vi "스테이트머신_계측기(간단).vi"() -> ()   [LabVIEW 2020]
panel:
  out "열거형":enum16{"초기", "대기", "계측"}(ring)
  out "진도":dbl(graph)
  in  "계측 시작":bool
  in  "프로그램 정지":bool
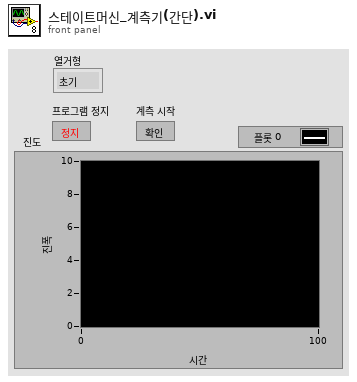
[diagram p1: front panel]
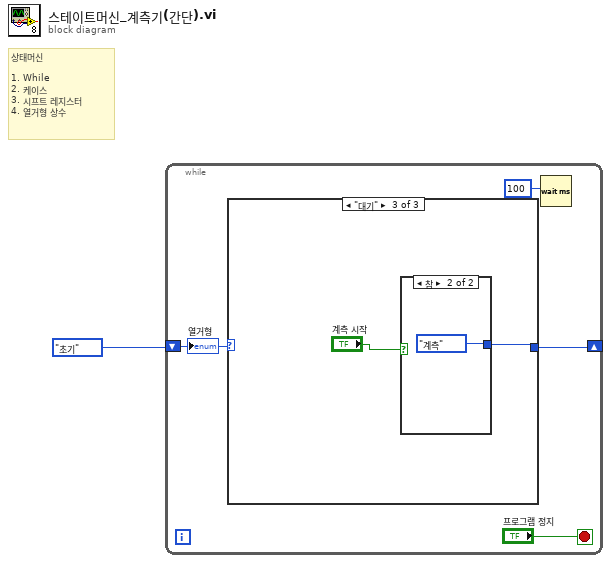
[diagram p0: block diagram]
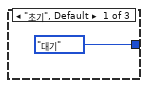
[diagram p2: hidden frame]
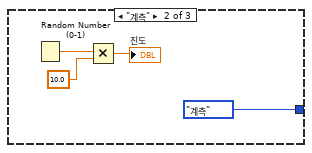
[diagram p3: hidden frame]
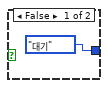
[diagram p4: hidden frame]
diagram:
  # "상태머신\n\n1. While\n2. 케이스 \n3. 시프트 레지스터\n4. 열거형 상수"
  n1 = while {
    shift-right: [w2] -> _
    shift-left: enum16{"초기", "대기", "계측"}."초기" -> [w4]
    stop <- "프로그램 정지" stop-if-true
    n2 = case shown="\"대기\"" w4 {
      tunnel: [enum16{"초기", "대기", "계측"}."대기" enum16{"초기", "대기", "계측"}."계측" w11] -> w2
      frame "초기", Default {
      }
      frame "계측" {
        n3 = Random Number (0-1)() -> (number: 0 to 1=w10:dbl)
        n4 = Multiply(x=w10, y=10.0) -> (x*y=→"진도":dbl)
      }
      frame "대기" {
        n5 = case shown="참" "계측 시작" {
          tunnel: [enum16{"초기", "대기", "계측"}."대기" enum16{"초기", "대기", "계측"}."계측"] -> w11
          frame False {
          }
          frame True {
          }
        }
      }
    }
    n6 = Wait (ms)(milliseconds to wait=u32 100 ("대기 시간 (ms)")) -> ()  [unwired: 1 out]
    "열거형" <- w4
  }
